vi "Read Title.vi"(8 "error in (no error)":errorcluster, 11 "Feed.lvclass in":refnum<class "Feed.lvclass">) -> (0 "error out":errorcluster, 2 "Title":string, 3 "Feed.lvclass out":refnum<class "Feed.lvclass">)   [LabVIEW 2017, in "Feed.lvclass"]
uses:
  <vilib>/NI_RSS/Feed/Feed.lvclass
  <vilib>/NI_RSS/Feed/Feed.lvclass/Feed.ctl
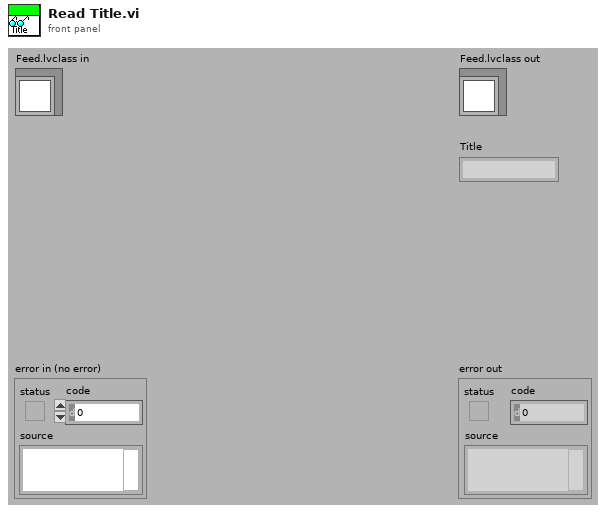
[diagram p1: front panel]
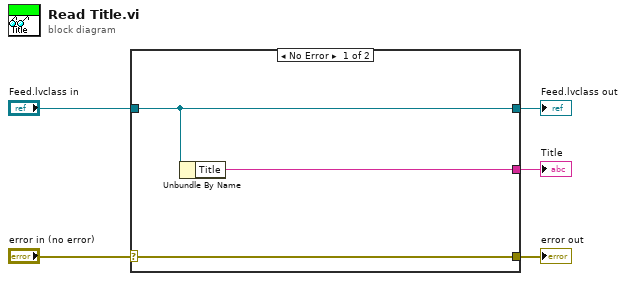
[diagram p0: block diagram]
diagram:
  n1 = case shown="No Error" "error in (no error)" {
    selector: "error in (no error)" -> [w8 w9]
    tunnel: [w8 w9] -> w4
    tunnel: [w7 w10] -> w2
    tunnel: "Feed.lvclass in" -> [w7 w10]
    tunnel: [w6 _] -> w1
    frame No Error {
      n2 = Unbundle By Name(w7) -> ("Title"=w6:string)
    }
    frame Error {
    }
  }
  "error out" <- w4
  "Feed.lvclass out" <- w2
  "Title" <- w1
